vi "Systemlink_Delete.vi"(10 "Tag Path":string, 11 "Device In":T1) -> ()   [LabVIEW 2016, in "Systemlink Tag.xctl"]
uses:
  Systemlink Tag.xctl
  SkylineCluster.ctl
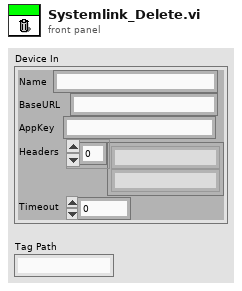
[diagram p1: front panel]
types:
  T1 = typedef "SkylineCluster.ctl" = cluster{"Name":string, "BaseURL":string, "AppKey":string, "Headers":string[], "Timeout":i32}
  T2 = enum16{"GET", "PUT", "POST", "MultiPOST", "DELETE"}
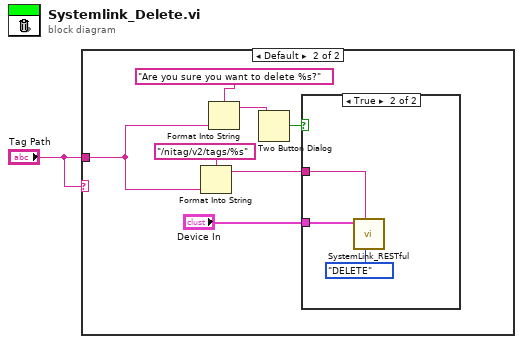
[diagram p0: block diagram]
diagram:
  n1 = case shown="Default" "Tag Path" {
    tunnel: "Tag Path" -> [_ w4]
    frame "" {
    }
    frame Default {
      n2 = Format Into String(format string="/nitag/v2/tags/%s" ("url"), w4) -> (resulting string=w8:string)  [unwired: 2 in, 1 out]
      n3 = Format Into String(format string="Are you sure you want to delete %s?" ("url"), w4) -> (resulting string=w3:string)  [unwired: 2 in, 1 out]
      n4 = Two Button Dialog(message=w3) -> (T button?=w2:bool)  [unwired: 2 in]
      n5 = case shown="True" w2 {
        tunnel: w8 -> [_ w11]
        tunnel: "Device In" -> [_ w10]
        frame False {
        }
        frame True {
          n6 = call "SystemLink_RESTful.vi"("Method"=T2."DELETE", "url"=w11, "Device In"=w10) -> ()  [unwired: 5 in, 4 out]
        }
      }
    }
  }
